vi "ConfigTrigger.vi"(8 "error in (no error)":errorcluster, 11 "HP3458aDMM in":refnum<class "HP3458aDMM.lvclass">) -> (0 "error out":errorcluster, 3 "HP3458aDMM out":refnum<class "HP3458aDMM.lvclass">)   [LabVIEW 2014, in "SamplerPlugins.lvlib" / "HP3458aDMM.lvclass"]
uses:
  HP3458aDMM.lvclass
  <vilib>/Utility/error.llb/Error Cluster From Error Code.vi
  <vilib>/ErrorRing/Error Ring.xnode
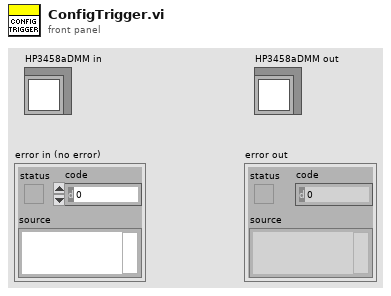
[diagram p1: front panel]
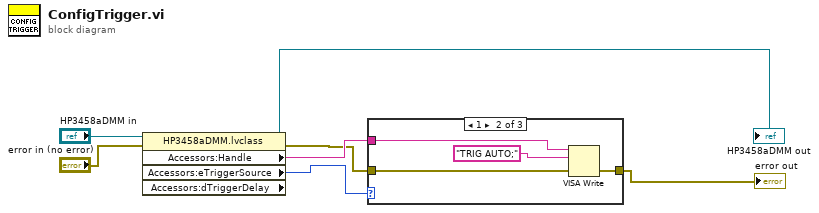
[diagram p0: block diagram]
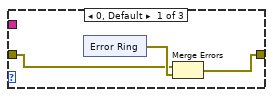
[diagram p2: hidden frame]
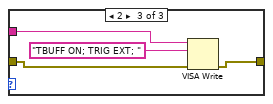
[diagram p3: hidden frame]
diagram:
  n1 = property class="HP3458aDMM.lvclass" props=["Accessors:Handle", "Accessors:eTriggerSource", "Accessors:dTriggerDelay"](reference="HP3458aDMM in", error in="error in (no error)") -> (reference out=→"HP3458aDMM out":refnum<class "HP3458aDMM.lvclass">, error out=w3:errorcluster, "Accessors:Handle"=w6:string, "Accessors:eTriggerSource"=w5:u16)  [unwired: 1 out]
  n2 = case shown="1" w5 {
    tunnel: w3 -> [w9 w18 w22]
    tunnel: [w8 w18 w19] -> w2
    tunnel: w6 -> [_ w16 w20]
    frame 0, Default {
      n3 = xnode "Error Ring"() -> ("error out"=w10:errorcluster)
      n4 = Merge Errors(w9, w10) -> (w8:errorcluster)
    }
    frame 1 {
      n5 = VISA Write(VISA resource name=w16, write buffer="TRIG AUTO;") -> ()  [unwired: 1 in, 3 out]
    }
    frame 2 {
      n6 = VISA Write(VISA resource name=w20, write buffer="TBUFF ON; TRIG EXT; ", error in (no error)=w22) -> (error out=w19:errorcluster)  [unwired: 2 out]
    }
  }
  "error out" <- w2
